vi "Main.vi"() -> ()   [LabVIEW 2026]
doc: "Illustre les principes de base du modèle de conception de machine à états dans LabVIEW. Les machines à états les plus simples sont composées d'une structure Condition dans une boucle While, avec un énum d'états câblé à un registre à décalage de la boucle pour définir l'exécution des différentes conditions (ou \"états\") de la structure Condition à différentes itérations de la boucle."
uses:
  SubVIs/Controls/Laser.ctl
  SubVIs/Controls/Etats.ctl
  SubVIs/Controls/TypeDef_FGV.ctl
panel:
  in  "Laser params":T1={"Emission (ON/OFF)"=FALSE, "Wavelength (nm)"=400.0, "Bandwidth (nm)"=10.0, "Power (%)"=0.0, "ND (%)"=0.0} {"ND (%)" min=0.0 max=100.0 step=1.0; "Power (%)" min=0.0 max=100.0 step=1.0; "Wavelength (nm)" min=400.0 max=840.0 step=10.0; "Bandwidth (nm)" min=10.0 max=100.0 step=10.0}
  out "error out":errorcluster caption="sortie d'erreur"
  in  "error in":errorcluster caption="entrée d'erreur"
  in  "Arrêter":bool
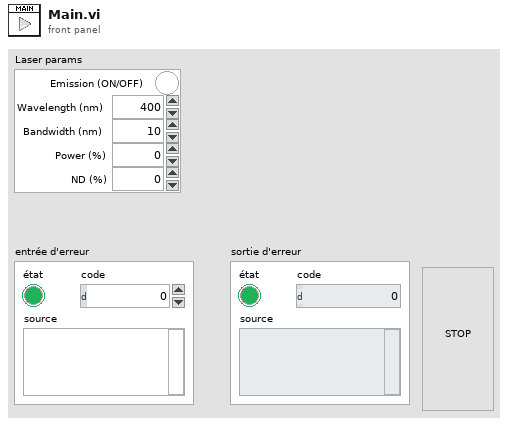
[diagram p1: front panel]
types:
  T1 = typedef "Laser.ctl" = cluster{"Emission (ON/OFF)":bool, "Wavelength (nm)":dbl, "Bandwidth (nm)":dbl, "Power (%)":dbl, "ND (%)":dbl}
  T2 = typedef "Etats.ctl" = enum16{"Init", "Stop", "Wait for Event", "Config"}
  T3 = typedef "TypeDef_FGV.ctl" = enum16{"Initialize", "Write", "Read"}
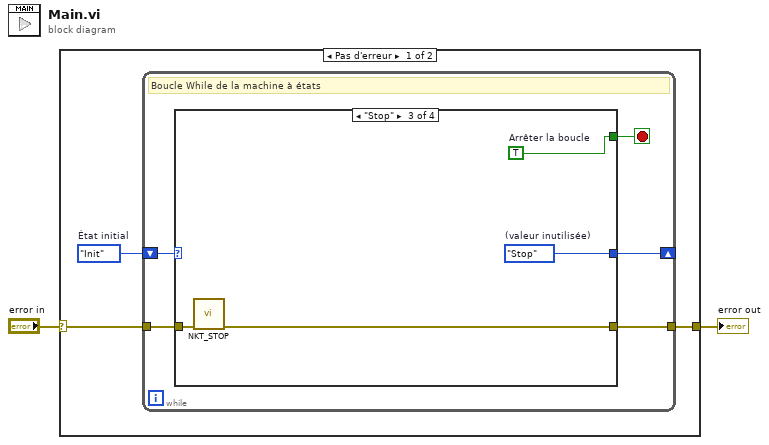
[diagram p0: block diagram]
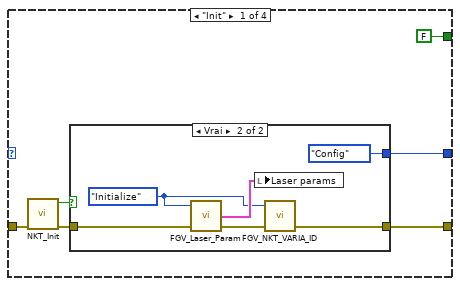
[diagram p2: hidden frame]
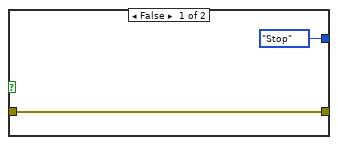
[diagram p3: hidden frame]
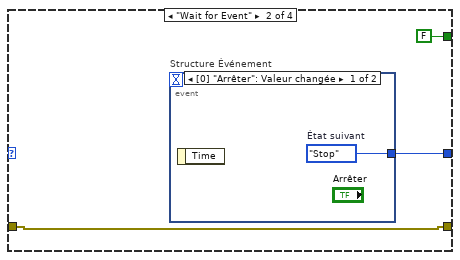
[diagram p4: hidden frame]
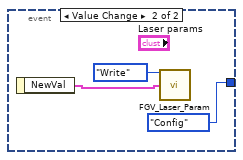
[diagram p5: hidden frame]
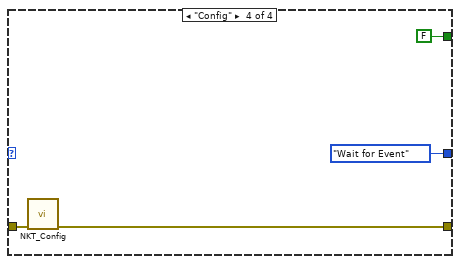
[diagram p6: hidden frame]
diagram:
  n1 = case shown="Pas d'erreur" "error in" {
    selector: "error in" -> [w4 w40]
    tunnel: [w3 w40] -> w1
    frame No Error {
      w5 = Etats."Init"  # État initial
      n2 = while {
        shift-right: [w9] -> _
        shift-left: w5 -> [w10]
        tunnel: w4 -> [w7]
        tunnel: [w6] -> w3
        stop <- w8 stop-if-true
        # "Boucle While de la machine à états"
        n3 = case "Structure Condition de machine à états" shown="\"Stop\"" w10 {
          tunnel: [w11 w27 w35 Etats."Wait for Event" ("(valeur inutilisée)")] -> w9
          tunnel: [FALSE ("Arrêter la boucle") FALSE ("Arrêter la boucle") w34 FALSE ("Arrêter la boucle")] -> w8
          tunnel: w7 -> [w15 w25 w33 w37]
          tunnel: [w13 w25 w32 w36] -> w6
          frame "Init" {
            # "Initialize - Dans cet exemple, la seule initialisation requise consiste à spécifier que l'état suivant de la machine à états est \"Wait for Event\"."
            n4 = call "NKT_Init.vi"("entrée d'erreur (pas d'erreur)"=w15) -> ("sortie d'erreur"=w14:errorcluster, "Found?"=w12:bool)  [unwired: 8 in, 1 out]
            n5 = case shown="Vrai" w12 {
              tunnel: w14 -> [w17 w24]
              tunnel: [w17 w20] -> w13
              tunnel: [Etats."Stop" ("État suivant") Etats."Config" ("État suivant")] -> w11
              frame False {
              }
              frame True {
                w19 = TypeDef_FGV."Initialize" ("Action")
                n6 = call "FGV_Laser_Param.vi"("error in"=w24, "Action"=w19) -> ("error out"=w21:errorcluster, "Laser params"=w23:T1)  [unwired: 2 in]
                n7 = local write "Laser params"(w23) -> ()
                n8 = call "FGV_NKT_VARIA_ID.vi"("error in"=w21, "Action"=w19) -> ("error out"=w20:errorcluster)  [unwired: 2 in, 1 out]
              }
            }
          }
          frame "Wait for Event" {
            n9 = event "Structure Événement" shown="[0] \"Arrêter\": Valeur changée" {
              selector: _ -> [_ _]
              dyn-events: _ -> [_ _]
              timeout: _ -> [_ _]
              tunnel: [w28 Etats."Config" ("État suivant")] -> w27
              event "Arrêter": Value Change {
                w28 = Etats."Stop"  # État suivant
                n10 = event-data() -> ()  [unwired: 1 in, 1 out]
              }
              event Value Change {
                n11 = event-data() -> ("NewVal"=w29:T1)  [unwired: 1 in]
                n12 = call "FGV_Laser_Param.vi"("Laser params"=w29, "Action"=TypeDef_FGV."Write") -> ()  [unwired: 2 in, 2 out]
              }
            }
          }
          frame "Stop" {
            w34 = TRUE  # Arrêter la boucle
            w35 = Etats."Stop"  # (valeur inutilisée)
            n13 = call "NKT_STOP.vi"("entrée d'erreur (pas d'erreur)"=w33) -> ("sortie d'erreur"=w32:errorcluster)  [unwired: 10 in]
          }
          frame "Config" {
            n14 = call "NKT_Config.vi"("entrée d'erreur (pas d'erreur)"=w37) -> ("sortie d'erreur"=w36:errorcluster)  [unwired: 10 in]
          }
        }
      }
    }
    frame Error {
    }
  }
  "error out" <- w1
